vi "Hub Read.vi"(4 "timeout ms (25000)":i32=250000, 6 "Bytes per sample":i32=4, 8 "error in (no error)":errorcluster, 9 "hub port":u64=2, 10 "Number of samples":u64, 11 "RP Instrument in":refnum<class "RP Instrument.lvclass">) -> (0 "error out":errorcluster, 2 "data out":string, 3 "RP Instrument out":refnum<class "RP Instrument.lvclass">)   [LabVIEW 2024, in "RP Instrument.lvclass"]
uses:
  RP Instrument.lvclass
  RP Instrument.lvclass/RP Instrument.ctl
  RP Communicator/RP Communicator.lvclass
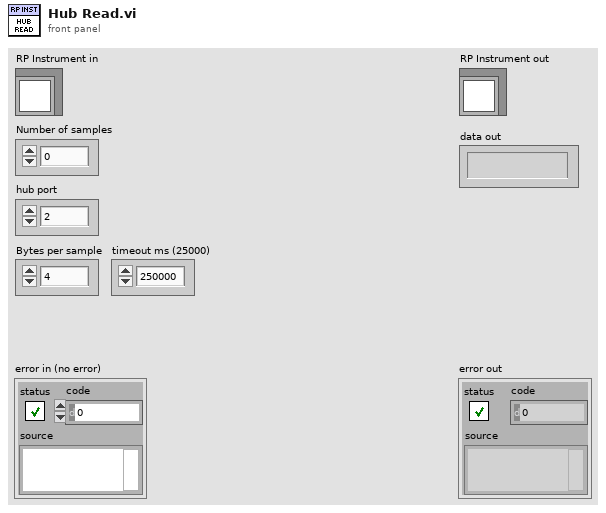
[diagram p1: front panel]
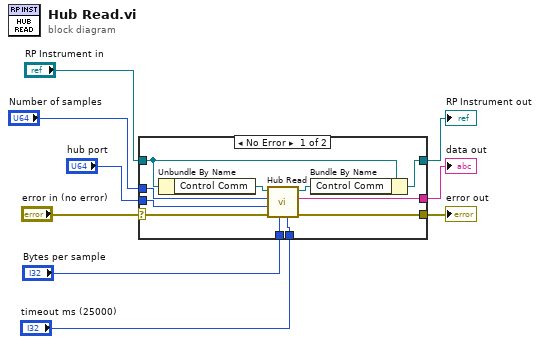
[diagram p0: block diagram]
diagram:
  n1 = case shown="No Error" "error in (no error)" {
    selector: "error in (no error)" -> [w18 w22]
    tunnel: [w17 w22] -> w8
    tunnel: [w16 w21] -> w6
    tunnel: "RP Instrument in" -> [w20 w21]
    tunnel: "Number of samples" -> [w14 _]
    tunnel: "hub port" -> [w13 _]
    tunnel: [w12 _] -> w3
    tunnel: "Bytes per sample" -> [w11 _]
    tunnel: "timeout ms (25000)" -> [w10 _]
    frame No Error {
      n2 = Unbundle By Name(w20) -> ("Control Comm"=w19:refnum<class "RP Communicator.lvclass">)
      n3 = call-dynamic "Hub Read.vi"("timeout ms (25000)"=w10, "Bytes per sample"=w11, "error in (no error)"=w18, "hub port"=w13, "Number of samples"=w14, "RP Communicator in"=w19) -> ("error out"=w17:errorcluster, "data out"=w12:string, "RP Communicator out"=w15:refnum<class "RP Communicator.lvclass">)  [unwired: 3 in]
      n4 = Bundle By Name(cluster=w20, "Control Comm"=w15) -> (w16:refnum<class "RP Instrument.lvclass">)
    }
    frame Error {
    }
  }
  "error out" <- w8
  "RP Instrument out" <- w6
  "data out" <- w3
